vi "Dequeue Message.vi"(8 "Error in":errorcluster, 11 "Queue Data in":T1) -> (0 "Error out":errorcluster, 1 "Data":variant, 2 "Cmd":string, 3 "Queue Data out":T1)   [LabVIEW 2018, in "Queue Messaging.lvlib"]
uses:
  Queue Messaging.lvlib
  QMH Template/Type Defs/EventsAndQueues--cluster.ctl
  Type Defs/Queue Message--cluster.ctl
  Event Messaging/Type Defs/Event Message--cluster.ctl
  QMH/QMH CORE.lvlib
  Event Messaging/Event Messaging.lvlib
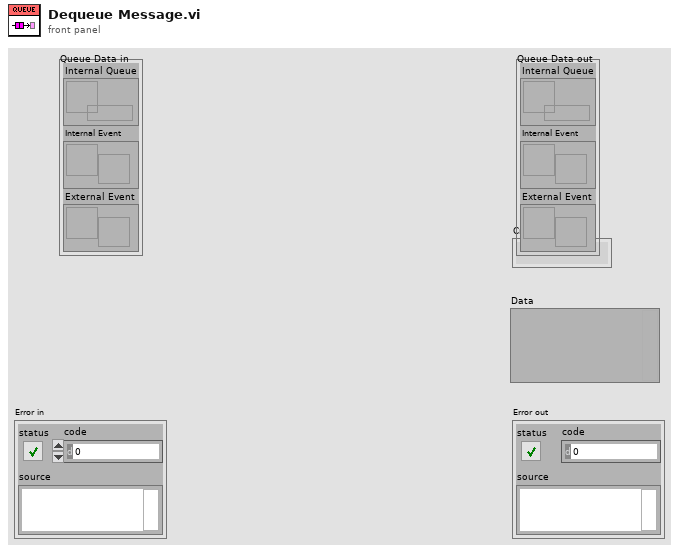
[diagram p1: front panel]
types:
  T1 = typedef "QMH CORE.lvlib/EventsAndQueues--cluster.ctl" = cluster{"Internal Queue":refnum<queue>, "Internal Event":refnum<user-event>, "External Event":refnum<user-event>}
  T2 = typedef "Queue Messaging.lvlib/Queue Message--cluster.ctl" = cluster{"Cmd":string, "Data":variant}
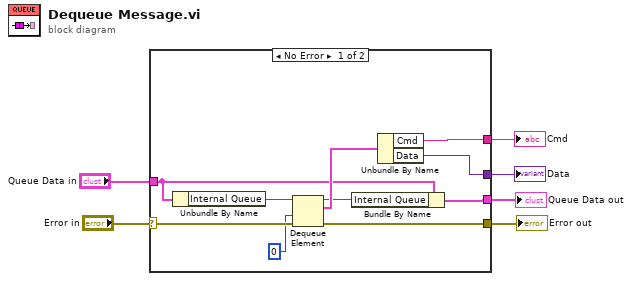
[diagram p0: block diagram]
diagram:
  n1 = case shown="No Error" "Error in" {
    selector: "Error in" -> [w16 w18]
    tunnel: [w7 w18] -> w5
    tunnel: [w14 _] -> w4
    tunnel: [w13 _] -> w3
    tunnel: "Queue Data in" -> [w9 w17]
    tunnel: [w10 w17] -> w1
    frame No Error {
      n2 = Unbundle By Name(w9) -> ("Internal Queue"=w12:refnum<queue>)
      n3 = Dequeue Element(queue=w12, timeout in ms (-1)=0, error in (no error)=w16) -> (queue out=w11:refnum<queue>, element=w15:T2, error out=w7:errorcluster)  [unwired: 1 out]
      n4 = Bundle By Name(cluster=w9, "Internal Queue"=w11) -> (w10:T1)
      n5 = Unbundle By Name(w15) -> ("Cmd"=w14:string, "Data"=w13:variant)
    }
    frame Error {
    }
  }
  "Error out" <- w5
  "Cmd" <- w4
  "Data" <- w3
  "Queue Data out" <- w1
